vi "Construct.vi"(6 "Bulk Size (1)":i32=1, 7 "Use system decimal point (F)":bool, 8 "error in (no error)":errorcluster, 9 "Constants":cluster{"name":string, "value":dbl}[](array[cluster]), 10 "Expression":string, 11 "Tag Expr in":refnum<class "Tag Expr.lvclass">) -> (0 "error out":errorcluster, 1 "error details":T1, 2 "Variable Names":string[](array[string]), 3 "Tag Expr out":refnum<class "Tag Expr.lvclass">)   [LabVIEW 2018, in "Tag Expr.lvclass"]
doc: "Construct a new muExpr instance. Input an expression or a set of expressions.\nReturns the expression handle and the list of variables found in the expression.\n\nOptionally input a list of constant name-value pairs.\n\nSet \"Use system decimal point\" to true if you want to adapt to the system's decimal point. If the system's decimal point is a comma, the argument separator will be changed to a semi-colon. The default decimal point is a period. The default argument separator is a comma.\n\nSet Bulk Size sets the range for bulk mode evaluations. Default is 1 (single result)."
uses:
  Tag Expr.lvclass
  Core/Tag Core.lvclass/Tag Core.ctl
  Tag/Tag.lvclass/Tag.ctl
  Tag Expr.lvclass/Tag Expr.ctl
  Tag/Read Type.vi
  Core/Get Tag LUT.vi
  <vilib>/Utility/error.llb/Error Cluster From Error Code.vi
  Tag/Tag.lvclass
  <vilib>/LAVA/muParser/mupExpr/mupExpr.lvclass
  Core/Tag Core.lvclass
panel:
  # "Construct a new muExpr instance. Input an expression or a set of expressions.\nReturns the expression handle and the list of variables found in the expression (for convenience)."
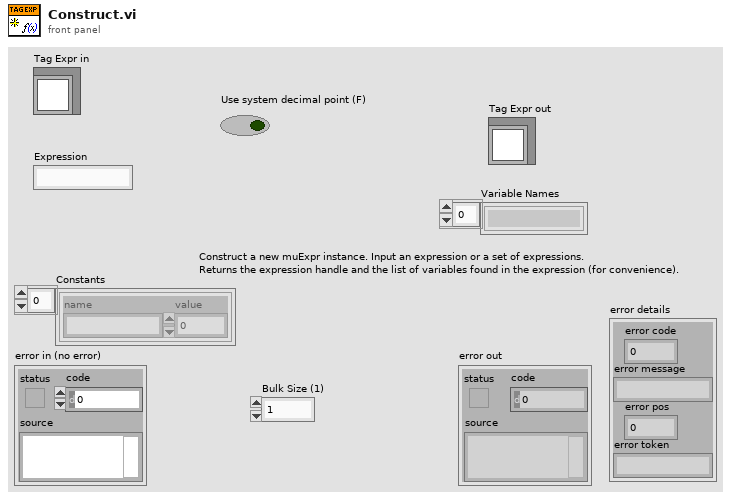
[diagram p1: front panel]
types:
  T1 = cluster{"error code":i32, "error message":string, "error pos":i32, "error token":string}
  T2 = typedef "NI_Data Type.lvlib/Data Type.ctl" = enum8{"Invalid Type", "Void", "I8", "I16", "I32", "I64", "U8", "U16", "U32", "U64", "Single Float", "Double Float", "Extended Float", "Single Complex", "Double Complex", "Extended Complex", "Enum U8", "Enum U16", "Enum U32", "Enum U64", "Single Float With Unit", "Double Float With Unit", "Extended Float With Unit", "Single Complex with Unit", "Double Complex with Unit", "Extended Complex with Unit", "Boolean", "String", "Path", "Picture", "Tag", "Array", "Cluster", "Variant", "LV Variant", "Waveform", "Timestamp", "Digital Waveform", "Digital Data", "ExpressData", "Refnum", "External Data", "VI", "Poly VI", "LabVIEW Class Instance", "Fixed Point"}
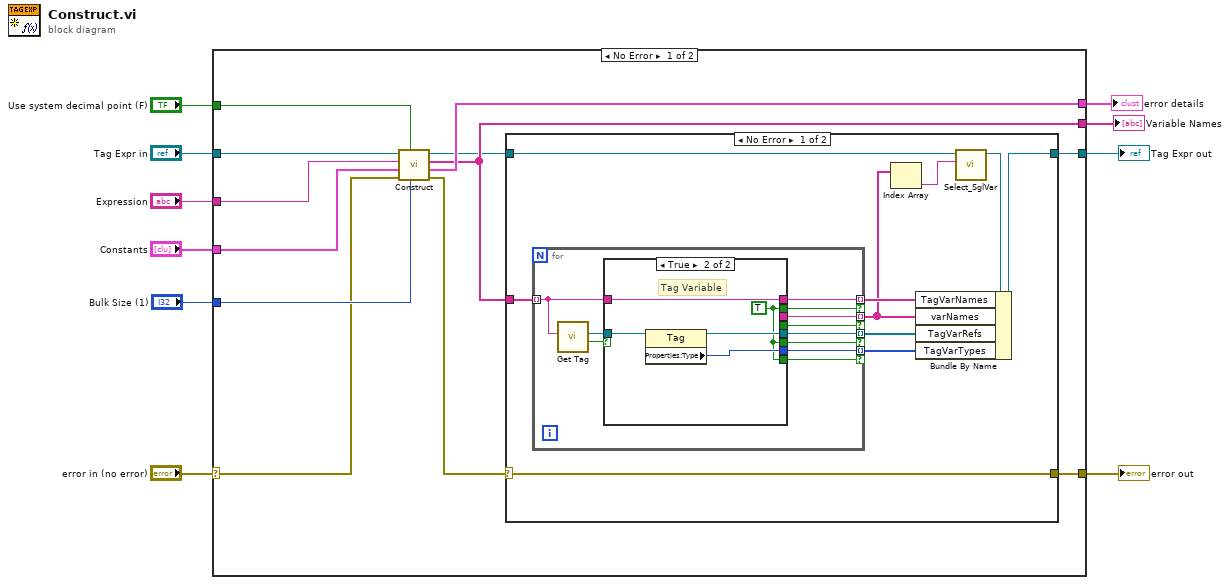
[diagram p0: block diagram]
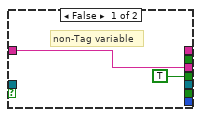
[diagram p2: hidden frame]
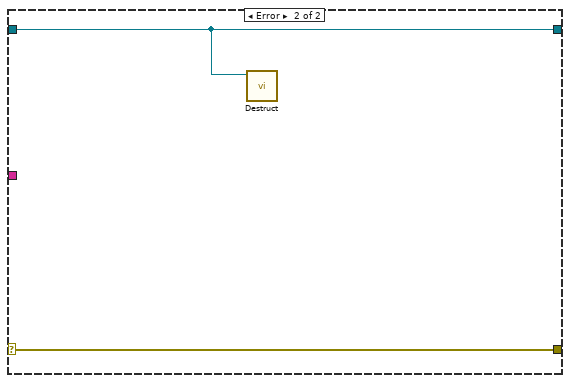
[diagram p3: hidden frame]
diagram:
  n1 = case shown="No Error" "error in (no error)" {
    selector: "error in (no error)" -> [w16 w53]
    tunnel: [w11 w53] -> w10
    tunnel: [w22 _] -> w9
    tunnel: [w15 _] -> w8
    tunnel: [w13 w54] -> w7
    tunnel: "Bulk Size (1)" -> [w21 _]
    tunnel: "Use system decimal point (F)" -> [w20 _]
    tunnel: "Constants" -> [w19 _]
    tunnel: "Expression" -> [w18 _]
    tunnel: "Tag Expr in" -> [w17 w54]
    frame No Error {
      n2 = call-parent "Construct.vi"("Bulk Size (1)"=w21, "Use system decimal point (F)"=w20, "error in (no error)"=w16, "Constants"=w19, "Expression"=w18, "muExpr in"=w17) -> ("error out"=w12:errorcluster, "error details"=w22:T1, "Variable Names"=w15:string[], "mupExpr out"=w14:refnum<class "Tag Expr.lvclass">)  [unwired: 2 in]
      n3 = case shown="No Error" w12 {
        selector: w12 -> [w30 w52]
        tunnel: w15 -> [w32 _]
        tunnel: w14 -> [w26 w51]
        tunnel: [w31 w51] -> w13
        tunnel: [w30 w52] -> w11
        frame No Error {
          n4 = for {
            tunnel: w32 -> [w41] mode=indexing
            tunnel: [w40] -> w29 mode=indexing if=w39
            tunnel: [w38] -> w24 mode=indexing if=w37
            tunnel: [w36] -> w28 mode=indexing if=w35
            tunnel: [w34] -> w27 mode=indexing if=w33
            n5 = call "Get Tag.vi"("Name"=w41) -> ("found"=w43:bool, "Tag Ref out"=w42:refnum<data-value>)  [unwired: 8 in, 1 out]
            n6 = case shown="True" w43 {
              tunnel: w42 -> [_ w49]
              tunnel: w41 -> [w45 w50]
              tunnel: [_ w50] -> w40
              tunnel: [_ w46] -> w39
              tunnel: [w45 _] -> w38
              tunnel: [TRUE _] -> w37
              tunnel: [_ w48] -> w36
              tunnel: [_ w46] -> w35
              tunnel: [_ w47] -> w34
              tunnel: [_ w46] -> w33
              frame False {
                # "non-Tag variable"
              }
              frame True {
                w46 = TRUE
                # "Tag Variable"
                n7 = property class="Tag"(reference=w49) -> (reference out=w48:refnum<data-value>, "Properties:Type"=w47:T2)  [unwired: 1 in, 1 out]
              }
            }
          }
          n8 = Index Array(array=w24) -> (element=w23:string)  [unwired: 1 in]
          n9 = call-dynamic "Select_SglVar.vi"("varName"=w23, "muExpr in"=w26) -> ("muExpr out"=w25:refnum<class "Tag Expr.lvclass">)  [unwired: 8 in, 1 out]
          n10 = Bundle By Name(cluster=w25, "TagVarNames"=w29, "varNames"=w24, "TagVarRefs"=w28, "TagVarTypes"=w27) -> (w31:refnum<class "Tag Expr.lvclass">)
        }
        frame Error {
          n11 = call-dynamic "Destruct.vi"("muExpr in"=w51) -> ()  [unwired: 10 in, 1 out]
        }
      }
    }
    frame Error {
    }
  }
  "error out" <- w10
  "Variable Names" <- w8
  "Tag Expr out" <- w7
  "error details" <- w9
